vi "AtlasLock.vi"(6 "LockStatus":string[](array[string]), 7 "Laser status":bool[](array[boolean]), 9 "Lock174":bool, 10 "Lock171":bool, 11 "Unlock":bool) -> ()   [LabVIEW 2017]
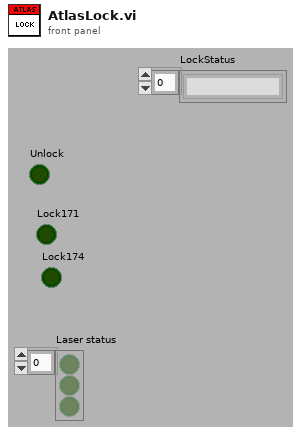
[diagram p1: front panel]
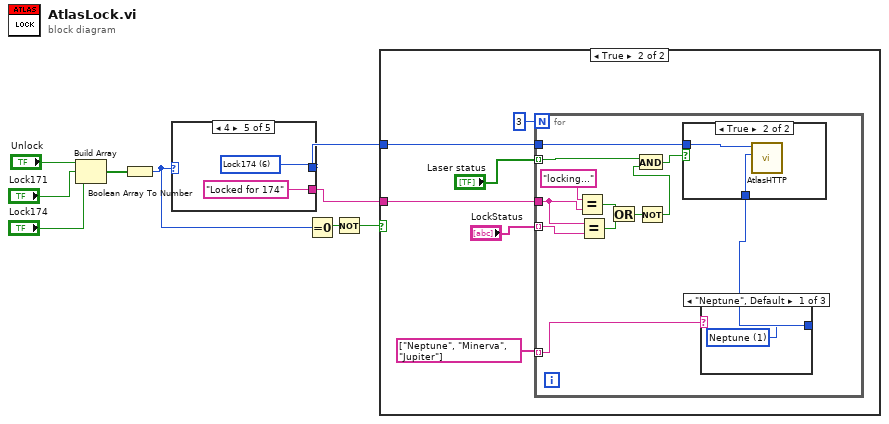
[diagram p0: block diagram]
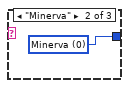
[diagram p4: hidden frame]
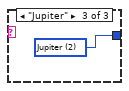
[diagram p5: hidden frame]
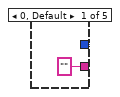
[diagram p6: hidden frame]
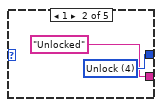
[diagram p7: hidden frame]
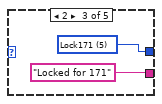
[diagram p8: hidden frame]
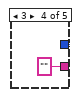
[diagram p9: hidden frame]
diagram:
  n1 = Build Array("Unlock", "Lock171", "Lock174") -> (w6:bool[])
  n2 = Boolean Array To Number(Boolean array=w6) -> (number=w4:u32)
  n3 = case shown="4" w4 {
    tunnel: [u16 0 ("Command") w13 w15 u16 0 ("Command") w19] -> w5
    tunnel: ["" "Unlocked" "Locked for 171" "" "Locked for 174"] -> w1
    frame 0, Default {
    }
    frame 1 {
      w13 = u16 4 items=["Login", "Logout", "get_laser_names", "Ping", "Unlock", "Lock171", "Lock174", "Connect", "Disconnect"] ("Command")
    }
    frame 2 {
      w15 = u16 5 items=["Login", "Logout", "get_laser_names", "Ping", "Unlock", "Lock171", "Lock174", "Connect", "Disconnect"] ("Command")
    }
    frame 3 {
    }
    frame 4 {
      w19 = u16 6 items=["Login", "Logout", "get_laser_names", "Ping", "Unlock", "Lock171", "Lock174", "Connect", "Disconnect"] ("Command")
    }
  }
  n4 = Equal To 0?(x=w4) -> (x = 0?=w3:bool)
  n5 = Not(x=w3) -> (.not. x?=w2:bool)
  n6 = case shown="True" w2 {
    tunnel: w5 -> [_ w24]
    tunnel: w1 -> [_ w21]
    frame False {
    }
    frame True {
      n7 = for {
        N: 3 -> [_]
        tunnel: string[] ["Neptune", "Minerva", "Jupiter"] -> [w37] mode=indexing
        tunnel: "Laser status" -> [w26] mode=indexing
        tunnel: w24 -> [w35]
        tunnel: w21 -> [w33]
        tunnel: "LockStatus" -> [w34] mode=indexing
        n8 = Equal?(x="locking...", y=w33) -> (x = y?=w31:bool)
        n9 = Equal?(x=w33, y=w34) -> (x = y?=w30:bool)
        n10 = Or(x=w31, y=w30) -> (x .or. y?=w29:bool)
        n11 = Not(x=w29) -> (.not. x?=w27:bool)
        n12 = And(x=w26, y=w27) -> (x .and. y?=w28:bool)
        n13 = case shown="\"Neptune\", Default" w37 {
          tunnel: [w40 w41 w42] -> w36
          frame "Neptune", Default {
            w40 = u16 1 items=["Minerva", "Neptune", "Jupiter"] ("Laser")
          }
          frame "Minerva" {
            w41 = u16 0 items=["Minerva", "Neptune", "Jupiter"] ("Laser")
          }
          frame "Jupiter" {
            w42 = u16 2 items=["Minerva", "Neptune", "Jupiter"] ("Laser")
          }
        }
        n14 = case shown="True" w28 {
          tunnel: w36 -> [_ w39]
          tunnel: w35 -> [_ w38]
          frame False {
          }
          frame True {
            n15 = call "AtlasHTTP.vi"("Laser"=w39, "Command"=w38) -> ()  [unwired: 6 in, 2 out]
          }
        }
      }
    }
  }
